vi "调整窗口.vi"(8 "error in (no error)":errorcluster caption="错误输入（无错误）", 10 "前面板范围":T1 caption="窗口范围", 11 "程序 输入":refnum<class "程序.lvclass">) -> (0 "error out":errorcluster caption="错误输出", 3 "程序 输出":refnum<class "程序.lvclass">)   [LabVIEW 2018, in "程序.lvclass"]
uses:
  <vilib>/Utility/miscctls.llb/LVRectTypeDef.ctl
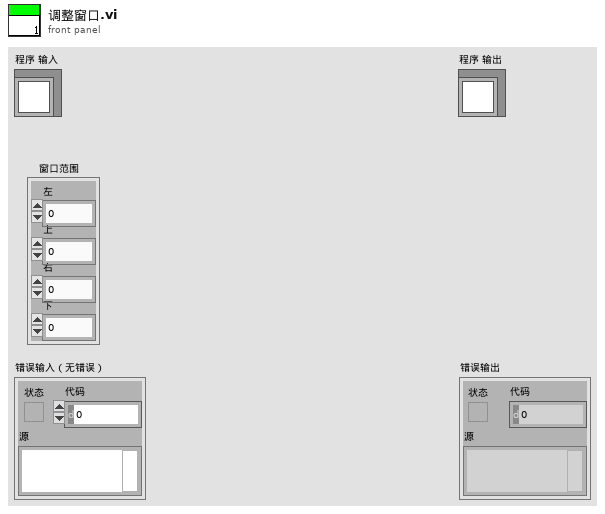
[diagram p1: front panel]
types:
  T1 = typedef "LVRectTypeDef.ctl" = cluster{"Left":i16, "Top":i16, "Right":i16, "Bottom":i16}
  T2 = typedef "LVBoundsTypeDef.ctl" = cluster{"Width":u32, "Height":u32}
  T3 = typedef "LVPositionTypeDef.ctl" = cluster{"Left":i32, "Top":i32}
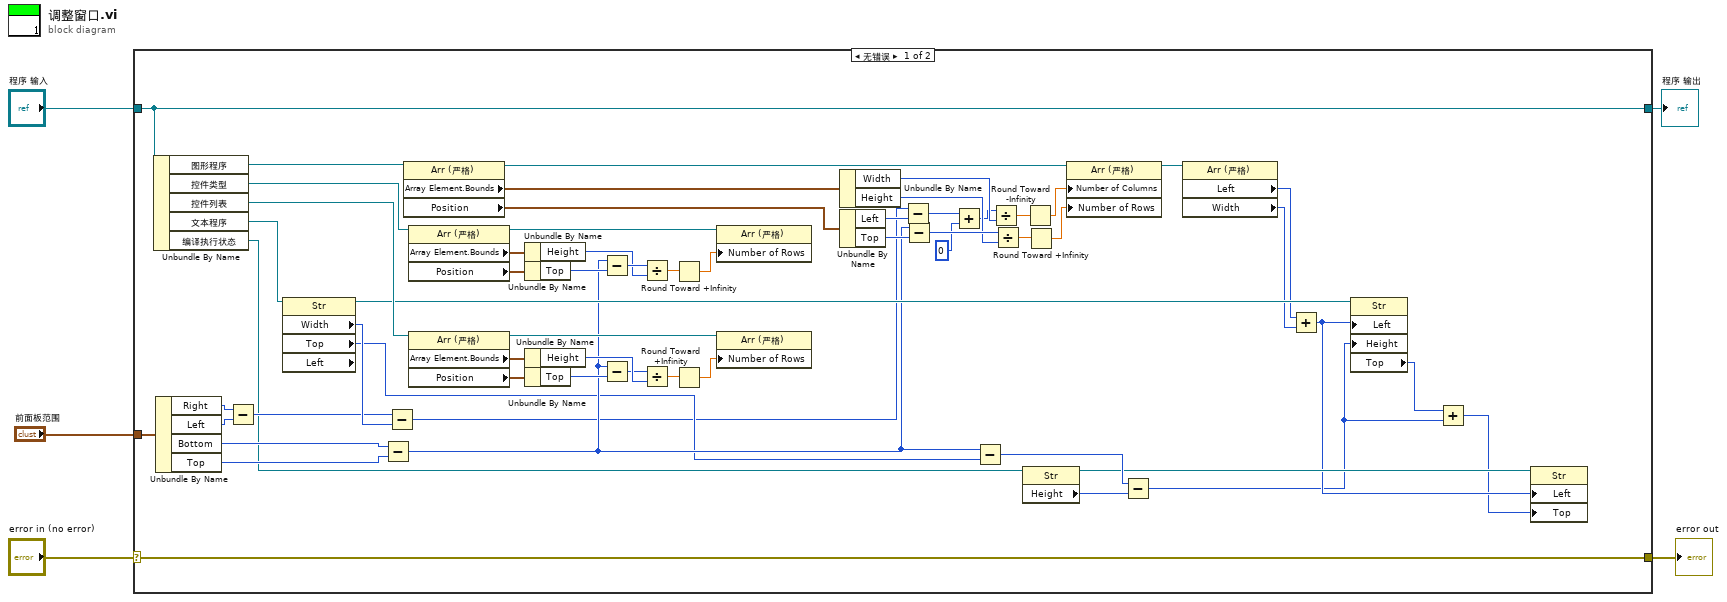
[diagram p0: block diagram]
diagram:
  n1 = case shown="无错误" "error in (no error)" {
    selector: "error in (no error)" -> [w64 w66]
    tunnel: [w64 w66] -> w4
    tunnel: [w63 w65] -> w2
    tunnel: "程序 输入" -> [w63 w65]
    tunnel: "前面板范围" -> [w61 _]
    frame No Error {
      n2 = Unbundle By Name(w63) -> ("图形程序"=w62:refnum<vi>, "控件类型"=w41:refnum<vi>, "控件列表"=w24:refnum<vi>, "文本程序"=w23:refnum<vi>, "编译执行状态"=w12:refnum<vi>)
      n3 = Unbundle By Name(w61) -> ("Right"=w60:i16, "Left"=w59:i16, "Bottom"=w58:i16, "Top"=w57:i16)
      n4 = Subtract(x=w60, y=w59) -> (x-y=w21:i16)
      n5 = property class="Str" props=["Width", "Top", "Left"](reference=w23) -> (reference out=w20:refnum<vi>, "Width"=w22:u32, "Top"=w15:i32)  [unwired: 1 in, 2 out]
      n6 = Subtract(x=w58, y=w57) -> (x-y=w16:i16)
      n7 = Subtract(x=w21, y=w22) -> (x-y=w14:u32)
      n8 = property class="Arr (严格)"(reference=w62) -> (reference out=w49:refnum<vi>, "Array Element.Bounds"=w53:T2, "Position"=w54:T3)  [unwired: 1 in, 1 out]
      n9 = property class="Arr (严格)"(reference=w41) -> (reference out=w34:refnum<vi>, "Array Element.Bounds"=w40:T2, "Position"=w39:T3)  [unwired: 1 in, 1 out]
      n10 = property class="Arr (严格)"(reference=w24) -> (reference out=w31:refnum<vi>, "Array Element.Bounds"=w25:T2, "Position"=w26:T3)  [unwired: 1 in, 1 out]
      n11 = Unbundle By Name(w40) -> ("Height"=w35:u32)
      n12 = Unbundle By Name(w39) -> ("Top"=w38:i32)
      n13 = Unbundle By Name(w25) -> ("Height"=w30:u32)
      n14 = Unbundle By Name(w26) -> ("Top"=w27:i32)
      n15 = Subtract(x=w16, y=w38) -> (x-y=w36:i32)
      n16 = Subtract(x=w16, y=w27) -> (x-y=w29:i32)
      n17 = Divide(x=w36, y=w35) -> (x/y=w37:dbl)
      n18 = Divide(x=w29, y=w30) -> (x/y=w28:dbl)
      n19 = Round Toward +Infinity(x=w37) -> (ceil(x): smallest int >= x=w33:dbl)
      n20 = Round Toward +Infinity(x=w28) -> (ceil(x): smallest int >= x=w32:dbl)
      n21 = property class="Arr (严格)"(reference=w34, "Number of Rows"=w33) -> ()  [unwired: 1 in, 2 out]
      n22 = property class="Arr (严格)"(reference=w31, "Number of Rows"=w32) -> ()  [unwired: 1 in, 2 out]
      n23 = Unbundle By Name(w53) -> ("Width"=w52:u32, "Height"=w50:u32)
      n24 = Unbundle By Name(w54) -> ("Left"=w56:i32, "Top"=w55:i32)
      n25 = Subtract(x=w14, y=w56) -> (x-y=w44:u32)
      n26 = Subtract(x=w16, y=w55) -> (x-y=w51:i32)
      n27 = Add(x=w44, y=0) -> (x+y=w43:u32)
      n28 = Subtract(x=w16, y=w15) -> (x-y=w13:i32)
      n29 = Divide(x=w43, y=w52) -> (x/y=w48:dbl)
      n30 = Divide(x=w51, y=w50) -> (x/y=w46:dbl)
      n31 = property class="Str"(reference=w12) -> (reference out=w10:refnum<vi>, "Height"=w11:u32)  [unwired: 1 in, 1 out]
      n32 = Round Toward -Infinity(1:w48) -> (0:w47:dbl)
      n33 = Round Toward +Infinity(x=w46) -> (ceil(x): smallest int >= x=w45:dbl)
      n34 = property class="Arr (严格)"(reference=w49, "Number of Columns"=w47, "Number of Rows"=w45) -> (reference out=w19:refnum<vi>)  [unwired: 1 in, 1 out]
      n35 = Subtract(x=w13, y=w11) -> (x-y=w7:u32)
      n36 = property class="Arr (严格)"(reference=w19) -> ("Left"=w18:i32, "Width"=w17:u32)  [unwired: 1 in, 2 out]
      n37 = Add(x=w18, y=w17) -> (x+y=w9:u32)
      n38 = property class="Str"(reference=w20, "Left"=w9, "Height"=w7) -> ("Top"=w8:i32)  [unwired: 1 in, 2 out]
      n39 = Add(x=w8, y=w7) -> (x+y=w6:u32)
      n40 = property class="Str"(reference=w10, "Left"=w9, "Top"=w6) -> ()  [unwired: 1 in, 2 out]
    }
    frame Error {
    }
  }
  "error out" <- w4
  "程序 输出" <- w2
